vi "Proportional Power BAP5.vi"(10 "Control Parameters":T1={"Setpoint"=50.0, "Control bandwidth"=4.0, "Settle bandwidth"=1.0, "Integral time"=30.0, "Int\non"=TRUE, "Derivative time"=0.5, "Der\non"=FALSE, "Settle time"=200.0} {"Settle time" format="%.2f"; "Derivative time" format="%.2f"; "Integral time" format="%.2f"; "Settle bandwidth" format="%.2f"; "Control bandwidth" format="%.2f"; "Setpoint" format="%.2f"}, 11 "Temp In (deg C)":dbl format="%.2f") -> (2 "Prop. Power":dbl format="%.2f")   [LabVIEW 2014]
doc: "Proportional Power BAP5\n\nCalculates normalized power based off of Current Temperature (°C), Setpoint (°C) ,and Control Bandwidth (°C).\n\nProportional Power = 0.5 - (Current Temp. / Setpoint), if this value is from 0 to 1.\n = 1, if this value is less than 0.\n = 0, if this value is greater than 1.\n\nBeverly Abadines \nPHY 350"
uses:
  typedefs/control parameters.ctl
panel:
  out "W/in control band?":bool
  # "Beverly Abadines\nPhys 350\nP5"
  # "Proportional Power"
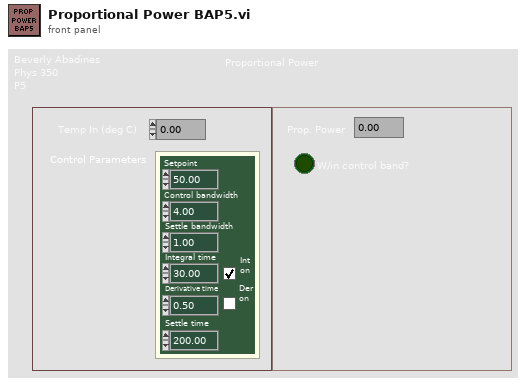
[diagram p1: front panel]
types:
  T1 = typedef "control parameters.ctl" = cluster{"Setpoint":dbl, "Control bandwidth":dbl, "Settle bandwidth":dbl, "Integral time":dbl, "Int\non":bool, "Derivative time":dbl, "Der\non":bool, "Settle time":dbl}
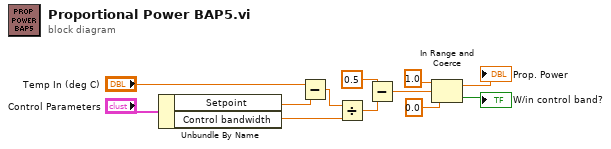
[diagram p0: block diagram]
diagram:
  n1 = Unbundle By Name("Control Parameters") -> ("Setpoint"=w8:dbl, "Control bandwidth"=w11:dbl)
  n2 = Subtract(x="Temp In (deg C)", y=w8) -> (x-y=w6:dbl)
  n3 = Divide(x=w6, y=w11) -> (x/y=w10:dbl)
  n4 = Subtract(x=0.5, y=w10) -> (x-y=w3:dbl)
  n5 = In Range and Coerce(upper limit=1.0, x=w3, lower limit=0.0) -> (coerced(x)=→"Prop. Power":dbl, In Range?=→"W/in control band?":bool)
